vi "Unflatten Value.vi"(8 "error in (no error)":errorcluster, 10 "Value":string, 11 "Boolean in":refnum<class "Assertion.lvclass">) -> (0 "error out":errorcluster, 3 "Boolean out":refnum<class "Assertion.lvclass">)   [LabVIEW 2019, in "Assertion.lvclass"]
uses:
  <vilib>/gpm_packages/@cs/data-type-serializer/source/Assertion/Assertion.lvclass
  <vilib>/gpm_packages/@cs/run-time-assertions/Source/Assert/Assert.lvclass
  <vilib>/gpm_packages/@cs/data-type-serializer/source/Assertion/Assertion.lvclass/Assertion.ctl
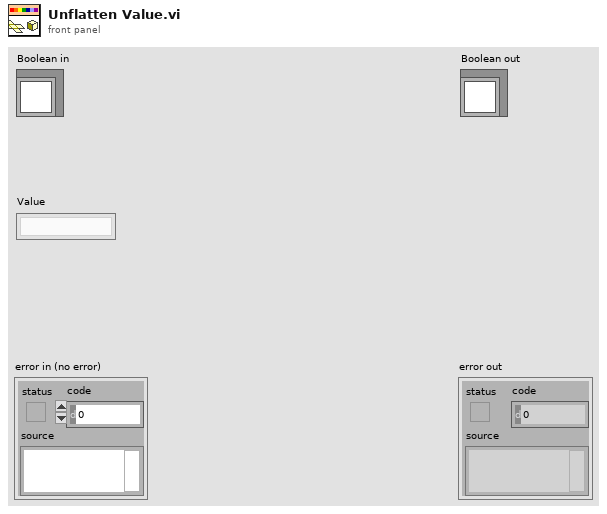
[diagram p1: front panel]
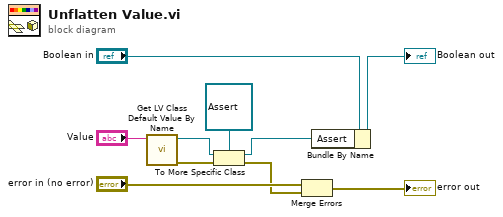
[diagram p0: block diagram]
diagram:
  n1 = call <vilib>:"Get LV Class Default Value By Name.vi"("class name"="Value") -> ("error out"=w5:errorcluster, "object"=w3:refnum<class>)  [unwired: 9 in]
  n2 = To More Specific Class(target class=refnum<class "Assert.lvclass"> refnum ("Assert"), reference=w3, error in=w5) -> (specific class reference=w1:refnum<class "Assert.lvclass">, error out=w4:errorcluster)
  n3 = Merge Errors("error in (no error)", w4) -> (→"error out":errorcluster)
  n4 = Bundle By Name(cluster="Boolean in", "Assert"=w1) -> (→"Boolean out":refnum<class "Assertion.lvclass">)
